vi "Load cluster config.vi"(10 "dup path":path, 11 "Test IN 2":T1={"Config HW"={"VISA Rigol DP832"="", "Config Rigol DP832"=[], "CTA Test#"="", "FT_Handle"=0, "Espera acceso FT"=0, "VISA Tek MDO3104"="Rigol_DP832", "VISA Key 81160A"="Rigol_DP832"}, "Config Test"=[], "Result"=[], "Execucion Test"={"Vasic Actual"=0}, "Config VGA"={"Theoretical Voltage"=[], "Real Voltage"=[], "Pulse Width"=0, "Frecuency Pulse"=0.0, "VGA Gain"=[]}, "Test Info"={"Asic"="", "Operator"="", "Place"="", "Time start"=timestamp(0 s since 1904-01-01), "Time stop"=timestamp(0 s since 1904-01-01)}, "Info machine"={"SO"="", "SO Name"="", "SO Ver"="", "SO Build"="", "CPU"="", "APP"="", "APP YEAR"="", "APP ver"="", "APP User"="", "APP Serail"="", "MAC"=[], "PC NAME"=[], "PC IP"=[], "BIOS MANU"="", "BIOS NAME"="", "BIOS SERIAL"="", "BOARD MANU"="", "BOARD NAME"="", "BOARD SERIAL"="", "Driver Version"="", "Library Version"="", "FPGA Ver"=0, "ID CTA board"=0, "LAST BOOT"="", "LABVIEW Ver"=0}, "Partial Report"="", "CONFIG GEN"=[]} {"CONFIG GEN"."Vasic Theorical" min=1.0 max=1000000.0 step=1.0 format="%#_6pV"; "CONFIG GEN"."Frequency" min=0.001 max=333000000.0 step=1000.0 format="%#_6pHz"; "CONFIG GEN"."Leading Edge Time" min=1e-09 max=1.0 step=1e-10 format="%#_6ps"; "CONFIG GEN"."Trailing Edge Time" min=1e-09 max=1.0 step=1e-10 format="%#_6ps"; "CONFIG GEN"."Delay" min=0.0 max=1.0 step=1e-12 format="%#_6ps"; "CONFIG GEN"."Trigger Level Sync" items=["ECL", "TTL"]; "CONFIG GEN"."Trigger Sync Out" items=["AB"=3, "B"=2, "A"=1, "None"=0]; "CONFIG GEN"."Load" min=1.0 max=1000000.0 step=1.0 format="%#_6p"; "CONFIG GEN"."DC Offset" min=-10.0 max=10.0 step=0.1 format="%#_6pV"; "CONFIG GEN"."Amplitude" min=0.05 max=5.0 step=0.001 format="%#_6pV"; "CONFIG GEN"."Width Time" min=1.5e-09 max=1.0 step=1e-10 format="%#_6ps"; "CONFIG GEN"."Channel" items=["Channel1"=1, "Channel2"=2]; "Config VGA"."Theoretical Voltage" format="%1.4f"; "Config VGA"."VGA Gain" format="%02x"; "Config VGA"."Frecuency Pulse" format="%0_2p"; "Config VGA"."Pulse Width" format="%04x"; "Config VGA"."Real Voltage" format="%1.5f"; "Config Test"."VALUE IBIAS" max=63 step=1; "Config Test"."Vasic real f.a." min=2.8 max=3.8 step=0.01 format="%.2g"; "Config Test"."Limits Rate Scan adders"."Low" format="%1.3f"; "Config Test"."Limits Rate Scan adders"."High" format="%1.3f"; "Config Test"."Limits ADC"."High" format="%1.4f"; "Config Test"."Limits ADC"."Low" format="%1.3f"; "Config Test"."Lim offset Dig"."Max Dig" format="%.3g"; "Config Test"."Lim Offset Analog"."Min Analog" format="%.3g"; "Config Test"."Lim Offset Analog"."Max Analog" format="%.3g"; "Config Test"."Limits Rate Scan"."Low" format="%1.4f"; "Config Test"."Limits Rate Scan"."High" format="%1.3f"; "Config Test"."Limits Max PN Min NP"."Min P Upper" format="%.3g"; "Config Test"."Limits Max PN Min NP"."Min P Lower" format="%.3g"; "Config Test"."Limits Max PN Min NP"."Max N Lower" format="%.3g"; "Config Test"."Limits Max PN Min NP"."Max N Upper" format="%.3g"; "Config Test"."Limits Max PN Min NP"."Min N Lower" format="%.3g"; "Config Test"."Limits Max PN Min NP"."Min N Upper" format="%.3g"; "Config Test"."Limits Max PN Min NP"."Max P Upper" format="%.3g"; "Config Test"."Limits Max PN Min NP"."Max P Lower" format="%.3g"; "Config Test"."Vasic" min=2.8 max=3.8 step=0.01 format="%.2g"; "Config HW"."Config Rigol DP832"."Channel" items=["+30V Channel 1", "+30V Channel 2", "+5V Channel 3"]; "Config HW"."Config Rigol DP832"."V Limit" format="%.1g"; "Config HW"."Config Rigol DP832"."I Limit" format="%.1g"; "Config HW"."Config Rigol DP832"."V Out" format="%.1g"; "Result"."Test Registros"."Read W/R" format="%04x"; "Result"."Test Registros"."Pattern W/R" format="%04x"; "Result"."Test Registros"."Read Default" format="%04x"; "Result"."Test Registros"."Pattern Default" format="%04x"}) -> (3 "Test IN":T1={"Config HW"={"VISA Rigol DP832"="", "Config Rigol DP832"=[], "CTA Test#"="", "FT_Handle"=0, "Espera acceso FT"=0, "VISA Tek MDO3104"="Rigol_DP832", "VISA Key 81160A"="Rigol_DP832"}, "Config Test"=[], "Result"=[], "Execucion Test"={"Vasic Actual"=0}, "Config VGA"={"Theoretical Voltage"=[], "Real Voltage"=[], "Pulse Width"=0, "Frecuency Pulse"=0.0, "VGA Gain"=[]}, "Test Info"={"Asic"="", "Operator"="", "Place"="", "Time start"=timestamp(0 s since 1904-01-01), "Time stop"=timestamp(0 s since 1904-01-01)}, "Info machine"={"SO"="", "SO Name"="", "SO Ver"="", "SO Build"="", "CPU"="", "APP"="", "APP YEAR"="", "APP ver"="", "APP User"="", "APP Serail"="", "MAC"=[], "PC NAME"=[], "PC IP"=[], "BIOS MANU"="", "BIOS NAME"="", "BIOS SERIAL"="", "BOARD MANU"="", "BOARD NAME"="", "BOARD SERIAL"="", "Driver Version"="", "Library Version"="", "FPGA Ver"=0, "ID CTA board"=0, "LAST BOOT"="", "LABVIEW Ver"=0}, "Partial Report"="", "CONFIG GEN"=[]} {"CONFIG GEN"."Vasic Theorical" min=1.0 max=1000000.0 step=1.0 format="%#_6pV"; "CONFIG GEN"."Frequency" min=0.001 max=333000000.0 step=1000.0 format="%#_6pHz"; "CONFIG GEN"."Leading Edge Time" min=1e-09 max=1.0 step=1e-10 format="%#_6ps"; "CONFIG GEN"."Trailing Edge Time" min=1e-09 max=1.0 step=1e-10 format="%#_6ps"; "CONFIG GEN"."Delay" min=0.0 max=1.0 step=1e-12 format="%#_6ps"; "CONFIG GEN"."Trigger Level Sync" items=["ECL", "TTL"]; "CONFIG GEN"."Trigger Sync Out" items=["AB"=3, "B"=2, "A"=1, "None"=0]; "CONFIG GEN"."Load" min=1.0 max=1000000.0 step=1.0 format="%#_6p"; "CONFIG GEN"."DC Offset" min=-10.0 max=10.0 step=0.1 format="%#_6pV"; "CONFIG GEN"."Amplitude" min=0.05 max=5.0 step=0.001 format="%#_6pV"; "CONFIG GEN"."Width Time" min=1.5e-09 max=1.0 step=1e-10 format="%#_6ps"; "CONFIG GEN"."Channel" items=["Channel1"=1, "Channel2"=2]; "Config VGA"."Theoretical Voltage" format="%1.4f"; "Config VGA"."VGA Gain" format="%02x"; "Config VGA"."Frecuency Pulse" format="%0_2p"; "Config VGA"."Pulse Width" format="%04x"; "Config VGA"."Real Voltage" format="%1.5f"; "Config Test"."VALUE IBIAS" max=63 step=1; "Config Test"."Vasic real f.a." min=2.8 max=3.8 step=0.01 format="%.2g"; "Config Test"."Limits Rate Scan adders"."Low" format="%1.3f"; "Config Test"."Limits Rate Scan adders"."High" format="%1.3f"; "Config Test"."Limits ADC"."High" format="%1.4f"; "Config Test"."Limits ADC"."Low" format="%1.3f"; "Config Test"."Lim offset Dig"."Max Dig" format="%.3g"; "Config Test"."Lim Offset Analog"."Min Analog" format="%.3g"; "Config Test"."Lim Offset Analog"."Max Analog" format="%.3g"; "Config Test"."Limits Rate Scan"."Low" format="%1.4f"; "Config Test"."Limits Rate Scan"."High" format="%1.3f"; "Config Test"."Limits Max PN Min NP"."Min P Upper" format="%.3g"; "Config Test"."Limits Max PN Min NP"."Min P Lower" format="%.3g"; "Config Test"."Limits Max PN Min NP"."Max N Lower" format="%.3g"; "Config Test"."Limits Max PN Min NP"."Max N Upper" format="%.3g"; "Config Test"."Limits Max PN Min NP"."Min N Lower" format="%.3g"; "Config Test"."Limits Max PN Min NP"."Min N Upper" format="%.3g"; "Config Test"."Limits Max PN Min NP"."Max P Upper" format="%.3g"; "Config Test"."Limits Max PN Min NP"."Max P Lower" format="%.3g"; "Config Test"."Vasic" min=2.8 max=3.8 step=0.01 format="%.2g"; "Config HW"."Config Rigol DP832"."Channel" items=["+30V Channel 1", "+30V Channel 2", "+5V Channel 3"]; "Config HW"."Config Rigol DP832"."V Limit" format="%.1g"; "Config HW"."Config Rigol DP832"."I Limit" format="%.1g"; "Config HW"."Config Rigol DP832"."V Out" format="%.1g"; "Result"."Test Registros"."Read W/R" format="%04x"; "Result"."Test Registros"."Pattern W/R" format="%04x"; "Result"."Test Registros"."Read Default" format="%04x"; "Result"."Test Registros"."Pattern Default" format="%04x"})   [LabVIEW 2019]
uses:
  Test.ctl
  TEST.TEST CONFIG HW.ctl
  Rigol DP832/DP832_Control Channels.ctl
  TEST.TEST CONFIG TEST MATRIZ.ctl
  TEST.TEST CONFIG TEST.ctl
  TEST.TEST RESULT.ctl
  test_result fvasic.ctl
  TEST.TEST EXECUTION TEST.ctl
  TEST.TEST CONFIG VGA.ctl
  TEST.TEST TEST INFO.ctl
  TEST.TEST INFO PC.ctl
  GenPulse_configurar.ctl
panel:
  # "Modo 2\nModo 3\nModo 4\nModo 2\nModo 3\nModo 4"
  # "Modo 2\nModo 3\nModo 4\nModo 2\nModo 3\nModo 4"
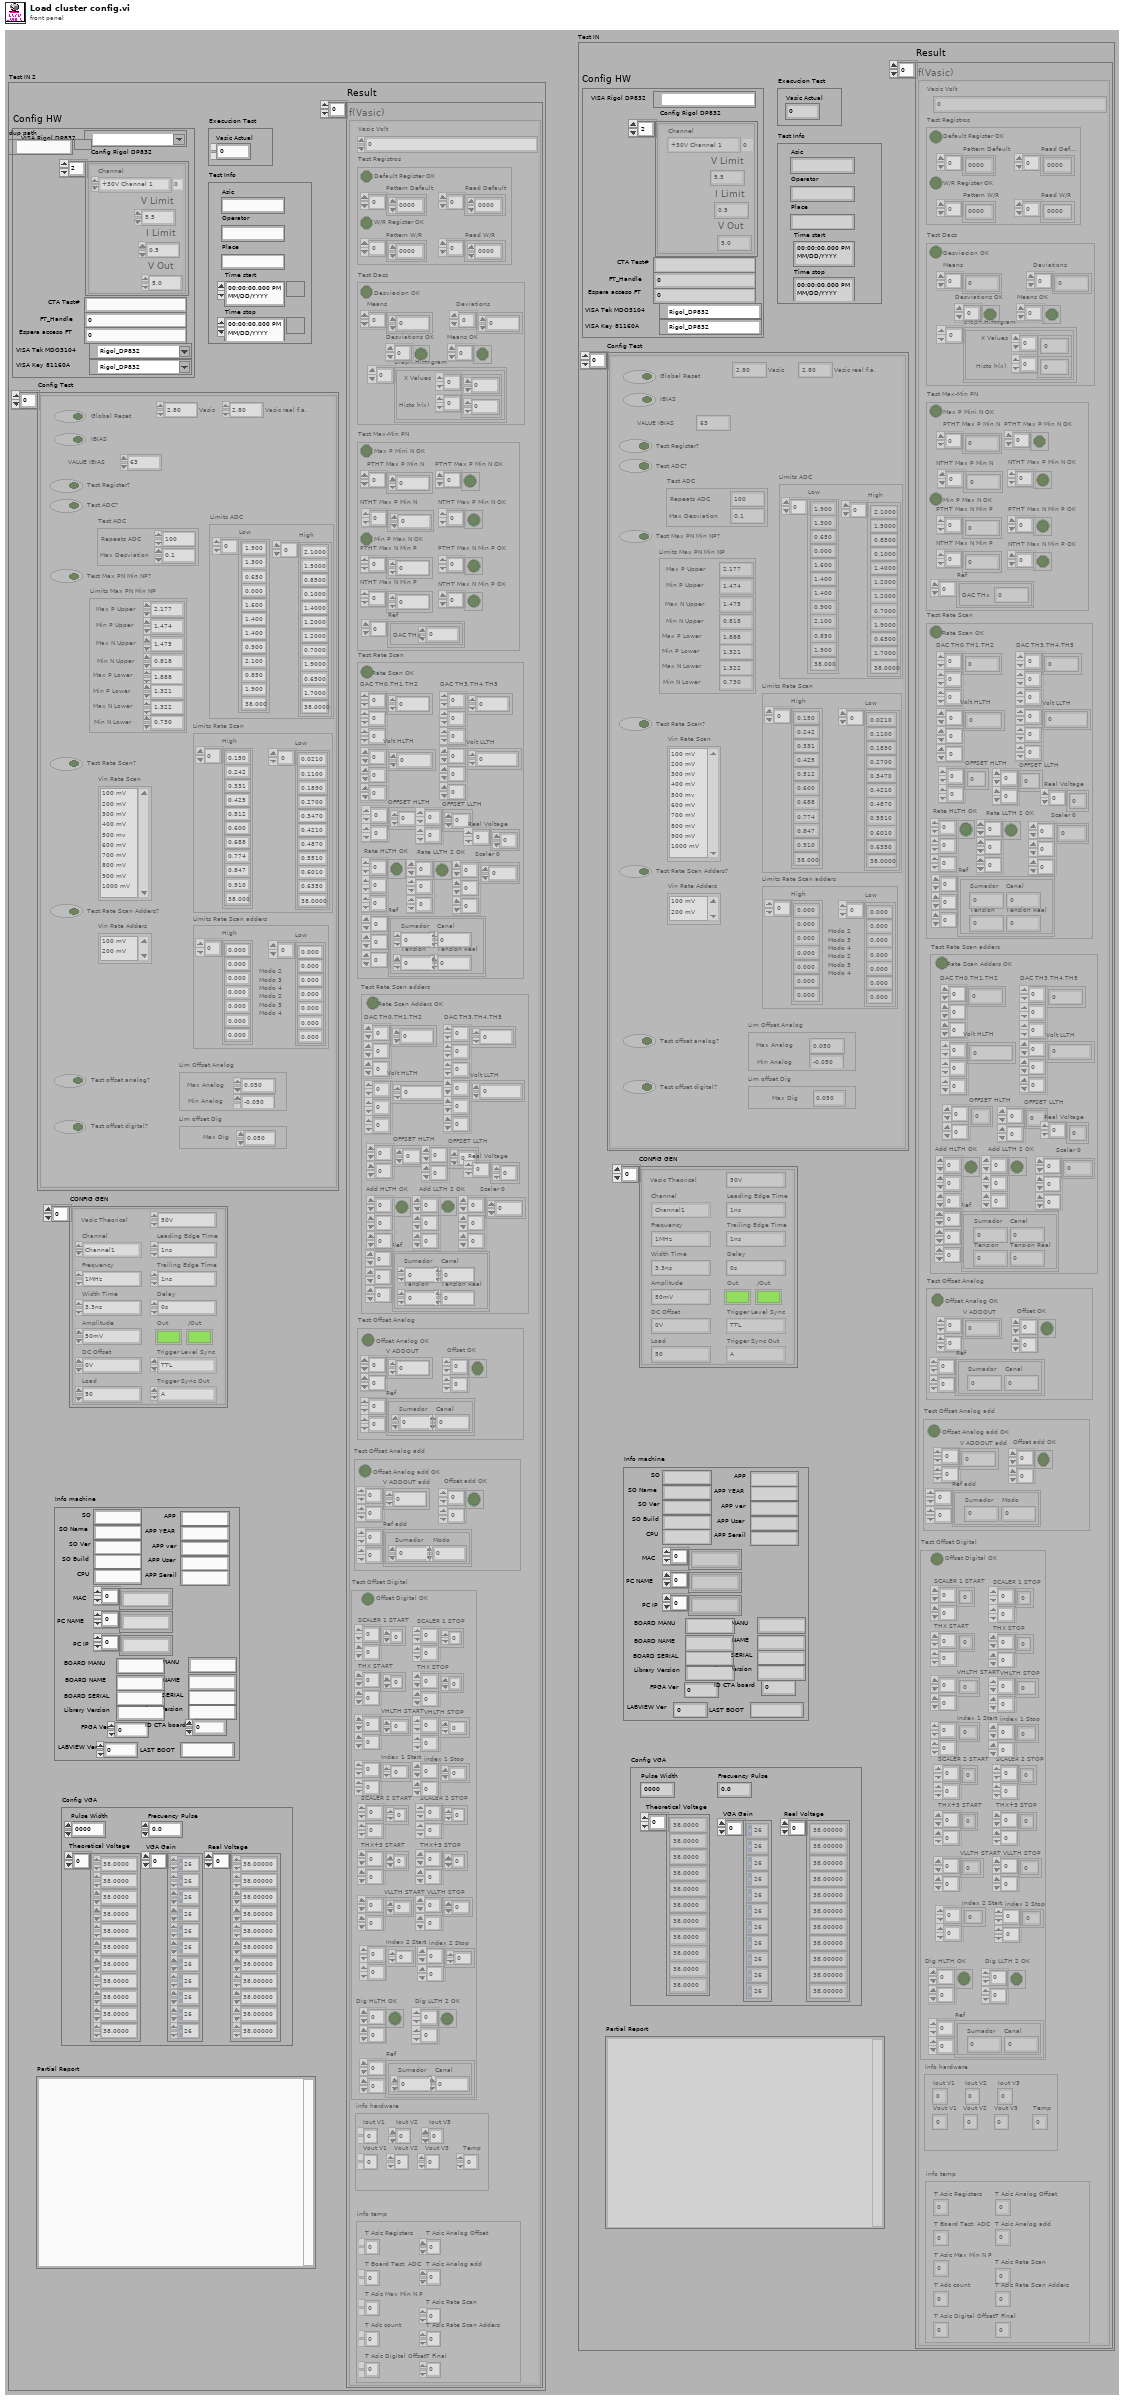
[diagram p1: front panel]
types:
  T1 = typedef "Test.ctl" = cluster{"Config HW":T2, "Config Test":T4, "Result":T6, "Execucion Test":T8, "Config VGA":T9, "Test Info":T10, "Info machine":T11, "Partial Report":string, "CONFIG GEN":T12[]}
  T2 = typedef "TEST.TEST CONFIG HW.ctl" = cluster{"VISA Rigol DP832":refnum<visa-resource-name>, "Config Rigol DP832":cluster{"Channel":T3, "V Limit":dbl, "I Limit":dbl, "V Out":dbl}[], "CTA Test#":string, "FT_Handle":u32, "Espera acceso FT":u32, "VISA Tek MDO3104":refnum<visa-resource-name>, "VISA Key 81160A":refnum<visa-resource-name>}
  T3 = typedef "DP832_Control Channels.ctl" = i32
  T4 = typedef "TEST.TEST CONFIG TEST MATRIZ.ctl" = T5[]
  T5 = typedef "TEST.TEST CONFIG TEST.ctl" = cluster{"Vasic":dbl, "Global Reset":bool, "Test Register?":bool, "Test ADC?":bool, "Test ADC":cluster{"Repeats ADC":i32, "Max Desviation":dbl}, "Limits ADC":cluster{"Low":dbl[], "High":dbl[]}, "Test Max PN Min NP?":bool, "Limits Max PN Min NP":cluster{"Max P Upper":dbl, "Min P Upper":dbl, "Max N Upper":dbl, "Min N Upper":dbl, "Max P Lower":dbl, "Min P Lower ":dbl, "Max N Lower":dbl, "Min N Lower":dbl}, "Test Rate Scan?":bool, "Vin Rate Scan":i32[], "Limits Rate Scan":cluster{"High":dbl[], "Low":dbl[]}, "Test Rate Scan Adders?":bool, "Vin Rate Adders":i32[], "Limits Rate Scan adders":cluster{"High":dbl[], "Low":dbl[]}, "Test offset analog?":bool, "Lim Offset Analog":cluster{"Max Analog":dbl, "Min Analog":dbl}, "Test offset digital?":bool, "Lim offset Dig":cluster{"Max Dig":dbl}, "Vasic real f.a.":dbl, "IBIAS":bool, "VALUE IBIAS":u8}
  T6 = typedef "TEST.TEST RESULT.ctl" = T7[]
  T7 = typedef "test_result fvasic.ctl" = cluster{"Vasic Volt":i32, "Test Registros":cluster{"Default Register OK":bool, "Pattern Default":u16[], "Read Default":u16[], "W/R Register OK":bool, "Pattern W/R":u16[], "Read W/R":u16[]}, "Test Dacs":cluster{"Desviacion OK":bool, "Means":dbl[], "Deviations":dbl[], "Desviations OK":bool[], "Means OK":bool[], "Graph Histogram":cluster{"X Values":dbl[], "Histo h(x)":i32[]}[]}, "Test Max-Min PN":cluster{"Max P Mini N OK":bool, "PTHT Max P Min N":dbl[], "PTHT Max P Min N OK":bool[], "NTHT Max P Min N":dbl[], "NTHT Max P Min N OK":bool[], "Min P Max N OK":bool, "PTHT Max N Min P":dbl[], "PTHT Max N Min P OK":bool[], "NTHT Max N Min P":dbl[], "NTHT Max N Min P OK":bool[], "Ref":cluster{"DAC THx":u8}[]}, "Test Rate Scan":cluster{"Rate Scan OK":bool, "DAC TH0,TH1,TH2":u16[][][], "Volt HLTH":dbl[][][], "Rate HLTH OK":bool[][][], "DAC TH3,TH4,TH5":u16[][][], "Volt LLTH":dbl[][][], "Rate LLTH 2 OK":bool[][][], "Scaler 0":u16[][][], "Ref":cluster{"Sumador":u8, "Canal":u8, "Tension":u8, "Tension Real":dbl}[][][], "OFFSET HLTH":dbl[][], "OFFSET LLTH":dbl[][], "Real Voltage":dbl[]}, "Test Rate Scan adders":cluster{"Rate Scan Adders OK":bool, "DAC TH0,TH1,TH2":u16[][][], "Volt HLTH":dbl[][][], "Add HLTH OK":bool[][][], "DAC TH3,TH4,TH5":u16[][][], "Volt LLTH":dbl[][][], "Add LLTH 2 OK":bool[][][], "Scaler 0":u16[][][], "Ref":cluster{"Sumador":u8, "Canal":u8, "Tension":u8, "Tension Real":dbl}[][][], "OFFSET HLTH":dbl[][], "OFFSET LLTH":dbl[][], "Real Voltage":dbl[]}, "Test Offset Analog":cluster{"Offset Analog OK":bool, "V ADDOUT":dbl[][], "Offset OK":bool[][], "Ref":cluster{"Sumador":u8, "Canal":u8}[][]}, "Test Offset Digital":cluster{"Offset Digital OK":bool, "SCALER 1 START":u16[][], "SCALER 1 STOP":u16[][], "THX START":u16[][], "THX STOP":u16[][], "VHLTH START":dbl[][], "VHLTH STOP":dbl[][], "Index 1 Start":i32[][], "index 1 Stop":i32[][], "SCALER 2 START":u16[][], "SCALER 2 STOP":u16[][], "THX+3 START":u16[][], "THX+3 STOP":u16[][], "VLLTH START":dbl[][], "VLLTH STOP":dbl[][], "Index 2 Start":i32[][], "index 2 Stop":i32[][], "Dig HLTH OK":bool[][], "Dig LLTH 2 OK":bool[][], "Ref":cluster{"Sumador":u8, "Canal":u8}[][]}, "info hardware":cluster{"Iout V1":dbl, "Iout V2":dbl, "Iout V3":dbl, "Vout V1":dbl, "Vout V2":dbl, "Vout V3":dbl, "Temp":dbl}, "Test Offset Analog add":cluster{"Offset Analog add OK":bool, "V ADDOUT add":dbl[][], "Offset add OK":bool[][], "Ref add":cluster{"Sumador":u8, "Modo":u8}[][]}, "info temp":cluster{"T Asic Registers":dbl, "T Board Test. ADC":dbl, "T Asic Max Min N P":dbl, "T Adc count":dbl, "T Asic Digital Offset":dbl, "T Asic Analog Offset":dbl, "T Asic Analog add":dbl, "T Asic Rate Scan":dbl, "T Asic Rate Scan Adders":dbl, "T Final":dbl}}
  T8 = typedef "TEST.TEST EXECUTION TEST.ctl" = cluster{"Vasic Actual":i32}
  T9 = typedef "TEST.TEST CONFIG VGA.ctl" = cluster{"Theoretical Voltage":dbl[], "Real Voltage":dbl[], "Pulse Width":u16, "Frecuency Pulse":dbl, "VGA Gain":u8[]}
  T10 = typedef "TEST.TEST TEST INFO.ctl" = cluster{"Asic":string, "Operator":string, "Place":string, "Time start":timestamp, "Time stop":timestamp}
  T11 = typedef "TEST.TEST INFO PC.ctl" = cluster{"SO":string, "SO Name":string, "SO Ver":string, "SO Build":string, "CPU":string, "APP":string, "APP YEAR":string, "APP ver":string, "APP User":string, "APP Serail":string, "MAC":string[], "PC NAME":string[], "PC IP":string[], "BIOS MANU":string, "BIOS NAME":string, "BIOS SERIAL":string, "BOARD MANU":string, "BOARD NAME":string, "BOARD SERIAL":string, "Driver Version":string, "Library Version":string, "FPGA Ver":u8, "ID CTA board":u64, "LAST BOOT":string, "LABVIEW Ver":u32}
  T12 = typedef "GenPulse_configurar.ctl" = cluster{"Channel":u16, "Frequency":dbl, "Width Time":dbl, "Amplitude":dbl, "DC Offset":dbl, "Load":dbl, "Leading Edge Time":dbl, "Trailing Edge Time":dbl, "Delay":dbl, "Out":bool, "/Out":bool, "Trigger Level Sync":u16, "Trigger Sync Out":u16, "Vasic Theorical":dbl}
  T13 = cluster{"Config HW":T2, "Config Test":T4, "Config VGA":T9, "CONFIG GEN":T12[]}
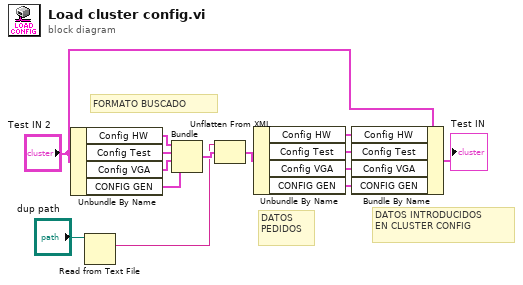
[diagram p0: block diagram]
diagram:
  # "DATOS INTRODUCIDOS\nEN CLUSTER CONFIG"
  # "DATOS\nPEDIDOS"
  # "FORMATO BUSCADO"
  n1 = Unbundle By Name("Test IN 2") -> ("Config HW"=w5:T2, "Config Test"=w6:T4, "Config VGA"=w7:T9, "CONFIG GEN"=w2:T12[])
  n2 = Read from Text File(file (use dialog)="dup path") -> (text=w4:string)  [unwired: 3 in, 3 out]
  n3 = Bundle("Config HW"=w5, "Config Test"=w6, "Config VGA"=w7, "CONFIG GEN"=w2) -> (w8:T13)  [unwired: 1 in]
  n4 = Unflatten From XML(xml string=w4, type=w8) -> (value=w11:T13)  [unwired: 1 in, 1 out]
  n5 = Unbundle By Name(w11) -> ("Config HW"=w12:T2, "Config Test"=w13:T4, "Config VGA"=w14:T9, "CONFIG GEN"=w1:T12[])
  n6 = Bundle By Name(cluster="Test IN 2", "Config HW"=w12, "Config Test"=w13, "Config VGA"=w14, "CONFIG GEN"=w1) -> (→"Test IN":T1)
